vi "svx_SC Line To FString.vi"(8 "trailing zeros":bool, 9 "Precision Type":u16(ring) items=["Digits of precision", "Significant digits"], 10 "Digits":u8=1, 11 "Type":i32(listbox)) -> (3 "format string":string)   [LabVIEW 2017, in "SVX SC Line.xctl"]
uses:
  <vilib>/addons/_XControls/Shaft Centerline/SVX SC Line.xctl
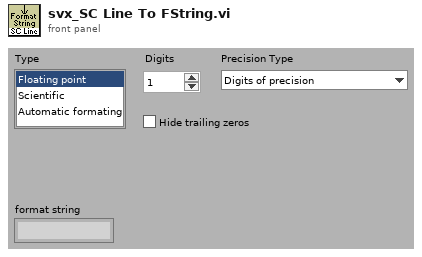
[diagram p1: front panel]
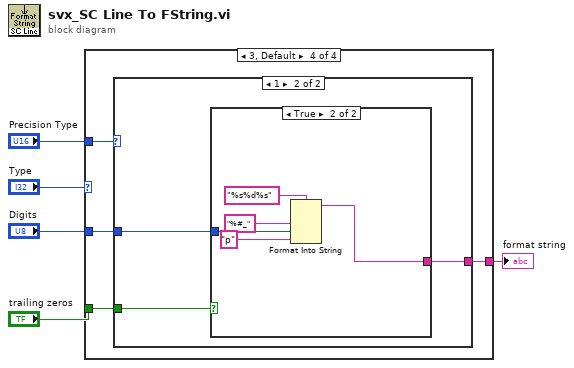
[diagram p0: block diagram]
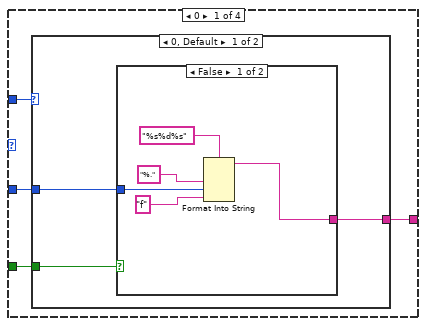
[diagram p2: hidden frame]
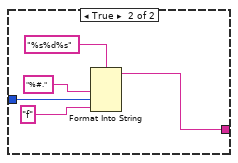
[diagram p3: hidden frame]
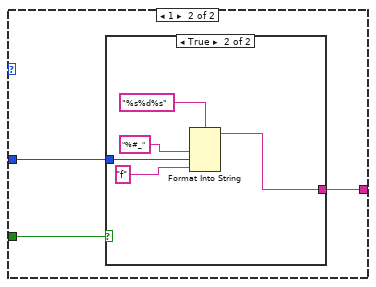
[diagram p4: hidden frame]
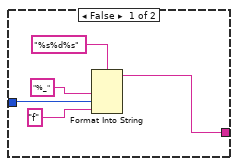
[diagram p5: hidden frame]
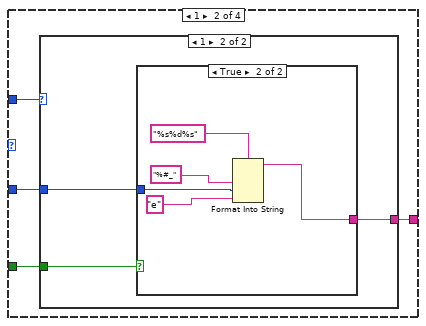
[diagram p6: hidden frame]
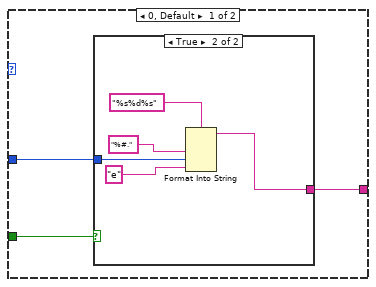
[diagram p7: hidden frame]
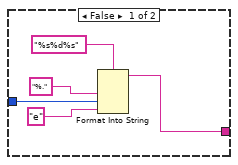
[diagram p8: hidden frame]
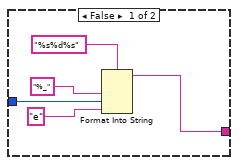
[diagram p9: hidden frame]
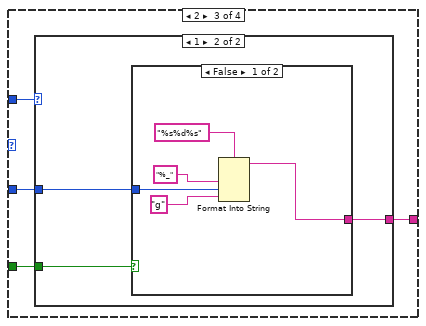
[diagram p10: hidden frame]
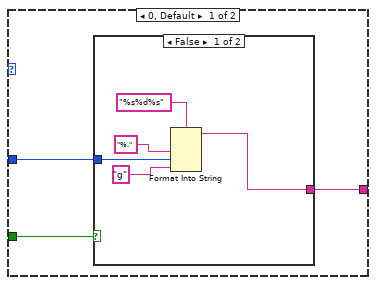
[diagram p11: hidden frame]
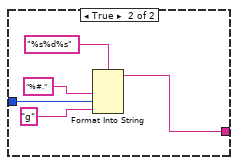
[diagram p12: hidden frame]
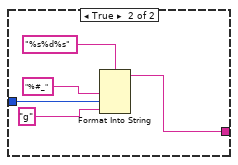
[diagram p13: hidden frame]
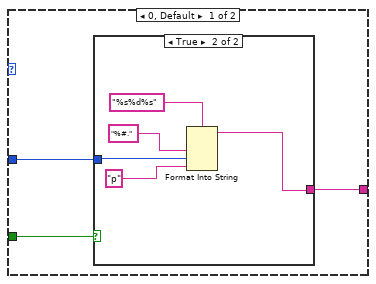
[diagram p14: hidden frame]
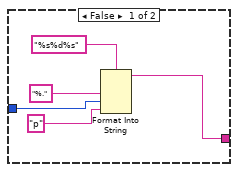
[diagram p15: hidden frame]
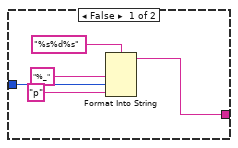
[diagram p16: hidden frame]
diagram:
  n1 = case shown="3, Default" "Type" {
    tunnel: "Precision Type" -> [w9 w36 w66 w96]
    tunnel: "trailing zeros" -> [w8 w37 w68 w98]
    tunnel: "Digits" -> [w7 w38 w67 w97]
    tunnel: [w6 w39 w69 w99] -> w1
    frame 0 {
      n2 = case shown="0, Default" w9 {
        tunnel: w8 -> [w12 w25]
        tunnel: w7 -> [w11 w23]
        tunnel: [w10 w24] -> w6
        frame 0, Default {
          n3 = case shown="False" w12 {
            tunnel: w11 -> [w16 w22]
            tunnel: [w14 w19] -> w10
            frame False {
              n4 = Format Into String(format string="%s%d%s", "%." ("input 1"), w16, "f" ("input 3")) -> (resulting string=w14:string)  [unwired: 2 in, 1 out]
            }
            frame True {
              n5 = Format Into String(format string="%s%d%s", "%#." ("input 1"), w22, "f" ("input 3")) -> (resulting string=w19:string)  [unwired: 2 in, 1 out]
            }
          }
        }
        frame 1 {
          n6 = case shown="True" w25 {
            tunnel: w23 -> [w30 w35]
            tunnel: [w26 w32] -> w24
            frame False {
              n7 = Format Into String(format string="%s%d%s", "%_" ("input 1"), w30, "f" ("input 3")) -> (resulting string=w26:string)  [unwired: 2 in, 1 out]
            }
            frame True {
              n8 = Format Into String(format string="%s%d%s", "%#_" ("input 1"), w35, "f" ("input 3")) -> (resulting string=w32:string)  [unwired: 2 in, 1 out]
            }
          }
        }
      }
    }
    frame 1 {
      n9 = case shown="1" w36 {
        tunnel: w37 -> [w42 w55]
        tunnel: w38 -> [w41 w53]
        tunnel: [w40 w54] -> w39
        frame 0, Default {
          n10 = case shown="True" w42 {
            tunnel: w41 -> [w47 w52]
            tunnel: [w44 w49] -> w40
            frame False {
              n11 = Format Into String(format string="%s%d%s", "%." ("input 1"), w47, "e" ("input 3")) -> (resulting string=w44:string)  [unwired: 2 in, 1 out]
            }
            frame True {
              n12 = Format Into String(format string="%s%d%s", "%#." ("input 1"), w52, "e" ("input 3")) -> (resulting string=w49:string)  [unwired: 2 in, 1 out]
            }
          }
        }
        frame 1 {
          n13 = case shown="True" w55 {
            tunnel: w53 -> [w60 w65]
            tunnel: [w57 w62] -> w54
            frame False {
              n14 = Format Into String(format string="%s%d%s", "%_" ("input 1"), w60, "e" ("input 3")) -> (resulting string=w57:string)  [unwired: 2 in, 1 out]
            }
            frame True {
              n15 = Format Into String(format string="%s%d%s", "%#_" ("input 1"), w65, "e" ("input 3")) -> (resulting string=w62:string)  [unwired: 2 in, 1 out]
            }
          }
        }
      }
    }
    frame 2 {
      n16 = case shown="1" w66 {
        tunnel: w68 -> [w72 w85]
        tunnel: w67 -> [w71 w83]
        tunnel: [w70 w84] -> w69
        frame 0, Default {
          n17 = case shown="False" w72 {
            tunnel: w71 -> [w77 w82]
            tunnel: [w74 w79] -> w70
            frame False {
              n18 = Format Into String(format string="%s%d%s", "%." ("input 1"), w77, "g" ("input 3")) -> (resulting string=w74:string)  [unwired: 2 in, 1 out]
            }
            frame True {
              n19 = Format Into String(format string="%s%d%s", "%#." ("input 1"), w82, "g" ("input 3")) -> (resulting string=w79:string)  [unwired: 2 in, 1 out]
            }
          }
        }
        frame 1 {
          n20 = case shown="False" w85 {
            tunnel: w83 -> [w90 w95]
            tunnel: [w87 w92] -> w84
            frame False {
              n21 = Format Into String(format string="%s%d%s", "%_" ("input 1"), w90, "g" ("input 3")) -> (resulting string=w87:string)  [unwired: 2 in, 1 out]
            }
            frame True {
              n22 = Format Into String(format string="%s%d%s", "%#_" ("input 1"), w95, "g" ("input 3")) -> (resulting string=w92:string)  [unwired: 2 in, 1 out]
            }
          }
        }
      }
    }
    frame 3, Default {
      n23 = case shown="1" w96 {
        tunnel: w98 -> [w102 w115]
        tunnel: w97 -> [w101 w113]
        tunnel: [w100 w114] -> w99
        frame 0, Default {
          n24 = case shown="True" w102 {
            tunnel: w101 -> [w106 w110]
            tunnel: [w103 w108] -> w100
            frame False {
              n25 = Format Into String(format string="%s%d%s", "%." ("input 1"), w106, "p" ("input 3")) -> (resulting string=w103:string)  [unwired: 2 in, 1 out]
            }
            frame True {
              n26 = Format Into String(format string="%s%d%s", "%#." ("input 1"), w110, "p" ("input 3")) -> (resulting string=w108:string)  [unwired: 2 in, 1 out]
            }
          }
        }
        frame 1 {
          n27 = case shown="True" w115 {
            tunnel: w113 -> [w120 w125]
            tunnel: [w117 w122] -> w114
            frame False {
              n28 = Format Into String(format string="%s%d%s", "%_" ("input 1"), w120, "p" ("input 3")) -> (resulting string=w117:string)  [unwired: 2 in, 1 out]
            }
            frame True {
              n29 = Format Into String(format string="%s%d%s", "%#_" ("input 1"), w125, "p" ("input 3")) -> (resulting string=w122:string)  [unwired: 2 in, 1 out]
            }
          }
        }
      }
    }
  }
  "format string" <- w1
